vi "SA_ATT.vi"(0 "Session In":refnum<visa-resource-name>="GPIB0::16::INSTR", 5 "ATT":dbl format="%#_13g", 7 "ATT":string, 11 "error in":errorcluster {"code" format="%.0x"}, 12 "RO (T)":bool) -> (4 "Session Out":refnum<visa-resource-name>, 8 "att":dbl, 14 "Ref LVL coerced (T)":bool, 15 "error out":errorcluster {"code" format="%.0x"})   [LabVIEW 2018]
doc: "Launches the Instrument I/O Assistant, which you can use to communicate with message-based instruments and graphically parse the response. For example you can communicate with an instrument that uses a serial, Ethernet, or GPIB interface."
panel:
  in  "Timeout":u32=3000
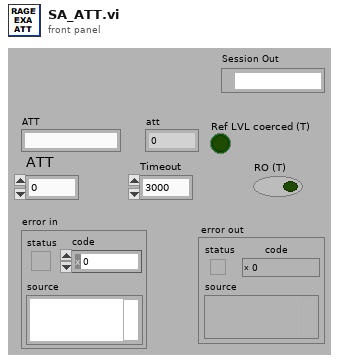
[diagram p1: front panel]
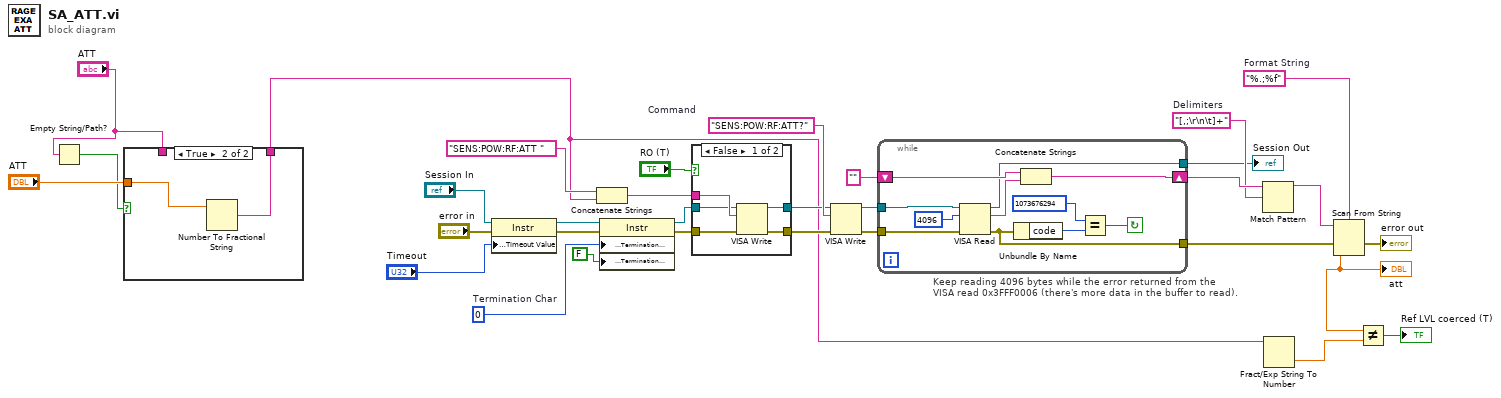
[diagram p0: block diagram]
diagram:
  w12 = "[,;\r\n\t]+"  # Delimiters
  w14 = "%.;%f"  # Format String
  w17 = "SENS:POW:RF:ATT?"  # Command
  w27 = u8 0  # Termination Char
  # "Keep reading 4096 bytes while the error returned from the\nVISA read 0x3FFF0006 (there's more data in the buffer to read)."
  n1 = Empty String/Path?(string/path="ATT") -> (empty?=w3:bool)
  n2 = case shown="True" w3 {
    tunnel: "ATT" -> [_ w35]
    tunnel: [w33 w34] -> w2
    tunnel: "ATT" -> [w33 _]
    frame False {
    }
    frame True {
      n3 = Number To Fractional String(number=w35) -> (F-format string=w34:string)  [unwired: 3 in]
    }
  }
  n4 = property class="Instr"(reference="Session In", error in="error in", "General Settings:Timeout Value"="Timeout") -> (reference out=w26:refnum<visa-resource-name>, error out=w29:errorcluster)
  n5 = Concatenate Strings("SENS:POW:RF:ATT " ("staticText"), w2) -> (w22:string)
  n6 = property class="Instr"(reference=w26, error in=w29, "Message Based Settings:Termination Character"=w27, "Message Based Settings:Termination Character Enable"=FALSE ("enable")) -> (reference out=w11:refnum<visa-resource-name>, error out=w28:errorcluster)
  n7 = case shown="False" "RO (T)" {
    tunnel: w28 -> [w40 w41]
    tunnel: [w39 w41] -> w23
    tunnel: w22 -> [w38 _]
    tunnel: w11 -> [w37 w42]
    tunnel: [w36 w42] -> w10
    frame False {
      n8 = VISA Write(VISA resource name=w37, write buffer=w38, error in (no error)=w40) -> (VISA resource name out=w36:refnum<visa-resource-name>, error out=w39:errorcluster)  [unwired: 1 out]
    }
    frame True {
    }
  }
  n9 = VISA Write(VISA resource name=w10, write buffer=w17, error in (no error)=w23) -> (VISA resource name out=w21:refnum<visa-resource-name>, error out=w20:errorcluster)  [unwired: 1 out]
  n10 = while {
    tunnel: w21 -> [w50]
    shift-right: [w44] -> w16
    shift-left: "" -> [w49]
    tunnel: w20 -> [w47]
    tunnel: [w46] -> w19
    tunnel: [w43] -> w9
    stop <- w45 continue-if-true
    n11 = VISA Read(VISA resource name=w50, byte count=u32 4096 ("byte count (0)"), error in (no error)=w47) -> (VISA resource name out=w43:refnum<visa-resource-name>, read buffer=w48:string, error out=w46:errorcluster)  [unwired: 1 out]
    n12 = Unbundle By Name(w46) -> ("code"=w52:i32)
    n13 = Concatenate Strings(w49, w48) -> (w44:string)
    n14 = Equal?(x=1073676294, y=w52) -> (x = y?=w45:bool)
  }
  "Session Out" <- w9
  n15 = Match Pattern(string=w16, regular expression=w12) -> (before substring=w15:string)  [unwired: 1 in, 3 out]
  n16 = Fract/Exp String To Number(string=w2) -> (number=w6:dbl)  [unwired: 3 in, 1 out]
  n17 = Scan From String(format string=w14, input string=w15, error in=w19) -> (error out=→"error out":errorcluster, output 1=w7:dbl)  [unwired: 2 in, 2 out]
  "att" <- w7
  n18 = Not Equal?(x=w7, y=w6) -> (x != y?=→"Ref LVL coerced (T)":bool)
